vi "test Print Entry with Sub-Entries.vi"(11 "Test Case In":refnum<class "test EDS.lvclass">) -> (0 "error out":errorcluster, 3 "Test Case Out":refnum<class "test EDS.lvclass">)   [LabVIEW 2024, in "test EDS.lvclass"]
uses:
  test EDS.lvclass
  Core/EDS/EDS.lvclass
  Core/EDS/EDS.lvclass/EDS.ctl
  <vilib>/Astemes/LUnit/Test Case.lvclass/Test Case.ctl
  2aee4a49-973f-4d4e-9175-22173d17c8e6.vi
  <vilib>/Astemes/LUnit/Append Pass Result.vi
  <vilib>/Astemes/LUnit/Append Fail Result.vi
  <vilib>/Astemes/LUnit/Describe Comparison.vi
  2aee4a49-973f-4d4e-9175-22173d17c8e6.vi/9c5d11cd-9439-4240-a1ee-d9baace9c924.vi
  <vilib>/Astemes/LUnit/Run In UI.vi
  <vilib>/Utility/error.llb/Clear Errors.vi
  <vilib>/Astemes/LUnit/Describe Variant.vi
  test EDS.lvclass/test EDS.ctl
  Core/Sorted Object Dictionary/Sorted Object Dictionary.lvclass
  Core/OD Entry/OD Entry.lvclass
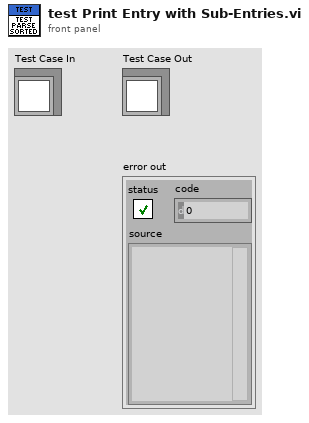
[diagram p1: front panel]
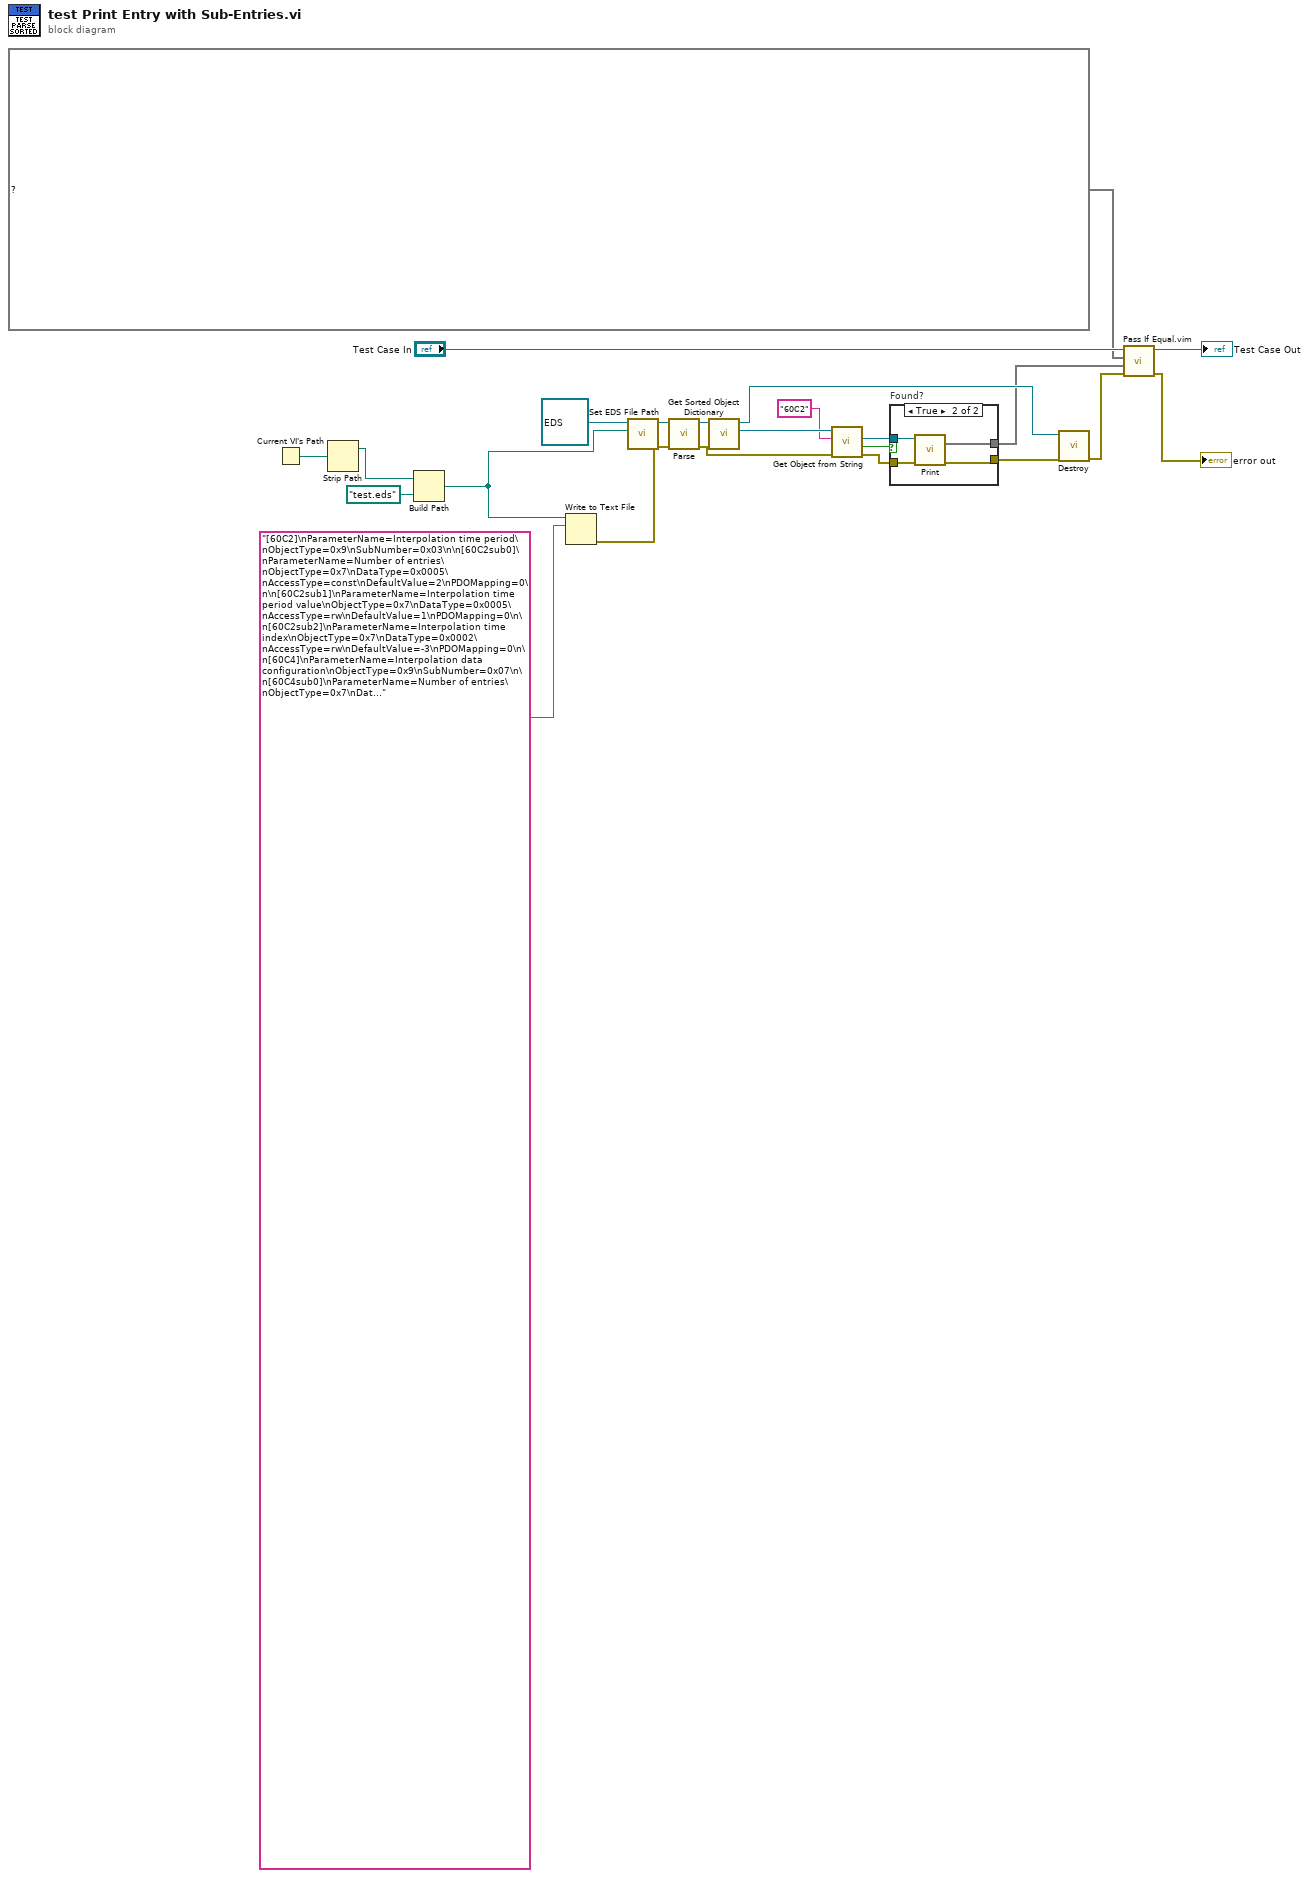
[diagram p0: block diagram]
diagram:
  n1 = Current VI's Path() -> (path=w18:path)
  n2 = Strip Path(path=w18) -> (stripped path=w14:path)  [unwired: 1 out]
  n3 = Build Path(base path=w14, name or relative path=path "test.eds") -> (appended path=w15:path)
  n4 = Write to Text File(file (use dialog)=w15, text="[60C2]\nParameterName=Interpolation time period\nObjectType=0x9\nSubNumber=0x03\n\n[60C2sub0]\nParameterName=Number of entries\nObjectType=0x7\nDataType=0x0005\nAccessType=const\nDefaultValue=2\nPDOMapping=0\n\n[60C2sub1]\nParameterName=Interpolation time period value\nObjectType=0x7\nDataType=0x0005\nAccessType=rw\nDefaultValue=1\nPDOMapping=0\n\n[60C2sub2]\nParameterName=Interpolation time index\nObjectType=0x7\nDataType=0x0002\nAccessType=rw\nDefaultValue=-3\nPDOMapping=0\n\n[60C4]\nParameterName=Interpolation data configuration\nObjectType=0x9\nSubNumber=0x07\n\n[60C4sub0]\nParameterName=Number of entries\nObjectType=0x7\nDataType=0x0005\nAccessType=const\nDefaultValue=6\nPDOMapping=0\n\n[60C4sub1]\nParameterName=MaximumBufferSize\nObjectType=0x7\nDataType=0x0007\nAccessType=ro\nDefaultValue=1\nPDOMapping=0\n\n[60C4sub2]\nParameterName=ActualBufferSize\nObjectType=0x7\nDataType=0x0007\nAccessType=rw\nDefaultValue=1\nPDOMapping=0\n\n[60C4sub3]\nParameterName=BufferOrganization\nObjectType=0x7\nDataType=0x0005\nAccessType=rw\nDefaultValue=0\nPDOMapping=0\n\n[60C4sub4]\nParameterName=BufferPosition\nObjectType=0x7\nDataType=0x0006\nAccessType=rw\nDefaultValue=1\nPDOMapping=0\n\n[60C4sub5]\nParameterName=SizeOfDataRecord\nObjectType=0x7\nDataType=0x0005\nAccessType=wo\nDefaultValue=4\nPDOMapping=0\n\n[60C4sub6]\nParameterName=BufferClear\nObjectType=0x7\nDataType=0x0005\nAccessType=wo\nDefaultValue=0\nPDOMapping=0") -> (error out=w16:errorcluster)  [unwired: 2 in, 2 out]
  n5 = call "Set EDS File Path.vi"("EDS File Path"=w15, "EDS in"=refnum<class "EDS.lvclass"> refnum ("EDS.lvlib:EDS.lvclass")) -> ("EDS out"=w19:refnum<class "EDS.lvclass">)  [unwired: 9 in]
  n6 = call "Parse.vi"("error in"=w16, "EDS in"=w19) -> ("error out"=w5:errorcluster, "EDS out"=w13:refnum<class "EDS.lvclass">)  [unwired: 8 in]
  n7 = call "Get Sorted Object Dictionary.vi"("EDS in"=w13) -> ("Sorted Object Dictionary"=w10:refnum<class "Sorted Object Dictionary.lvclass">, "EDS out"=w12:refnum<class "EDS.lvclass">)  [unwired: 9 in]
  n8 = call "Get Object from String.vi"("error in"=w5, "Index"="60C2", "Sorted Object Dictionary in"=w10) -> ("error out"=w4:errorcluster, "Found?"=w7:bool, "OD Entry"=w6:refnum<class "OD Entry.lvclass">)  [unwired: 5 in, 1 out]
  n9 = case "Found?" shown="True" w7 {
    tunnel: w6 -> [_ w28]
    tunnel: w4 -> [w24 w27]
    tunnel: [w24 w26] -> w8
    tunnel: [_ w25] -> w2
    frame False {
    }
    frame True {
      n10 = call "Print.vi"("error in"=w27, "OD Entry in"=w28) -> ("error out"=w26:errorcluster, "Entry with Sub-Entries"=w25:map{string, string}[])  [unwired: 7 in, 1 out]
    }
  }
  n11 = call "Destroy.vi"("error in"=w8, "EDS in"=w12) -> ("error out"=w9:errorcluster)  [unwired: 8 in, 1 out]
  n12 = call "Pass If Equal.vim"("error in (no error)"=w9, "Actual"=w2, "Expected"=map{string, string}[] [{"AccessType"="const", "CompactSubObj"="0", "DataType"="", "DefaultValue"="", "HighLimit"="", "Index"="0x60C2", "LowLimit"="", "ObjFlags"="0", "ObjectType"="RECORD", "PDOMapping"="0", "ParameterName"="Interpolation time period", "SubNumber"="3"}, {"AccessType"="const", "CompactSubObj"="0", "DataType"="UNSIGNED8", "DefaultValue"="2", "HighLimit"="", "Index"="0x00", "LowLimit"="", "ObjFlags"="0", "ObjectType"="VAR", "PDOMapping"="0", "ParameterName"="Number of entries", "SubNumber"=""}, {"AccessType"="rw", "CompactSubObj"="0", "DataType"="UNSIGNED8", "DefaultValue"="1", "HighLimit"="", "Index"="0x01", "LowLimit"="", "ObjFlags"="0", "ObjectType"="VAR", "PDOMapping"="0", "ParameterName"="Interpolation time period value", "SubNumber"=""}, {"AccessType"="rw", "CompactSubObj"="0", "DataType"="INTEGER8", "DefaultValue"="-3", "HighLimit"="", "Index"="0x02", "LowLimit"="", "ObjFlags"="0", "ObjectType"="VAR", "PDOMapping"="0", "ParameterName"="Interpolation time index", "SubNumber"=""}] ("Entry with Sub-Entries"), "LUnit Test Case In"="Test Case In") -> ("error out"=→"error out":errorcluster, "LUnit Test Case Out"=→"Test Case Out":refnum<class "test EDS.lvclass">)  [unwired: 6 in]
